vi "Write Result.vi"(8 "error in (no error)":errorcluster, 10 "Result":dbl, 11 "DBL Result Class in":refnum<class "DBL Result Class.lvclass">) -> (0 "error out":errorcluster, 3 "DBL Result Class out":refnum<class "DBL Result Class.lvclass">)   [LabVIEW 2018, in "DBL Result Class.lvclass"]
uses:
  DBL Result Class.lvclass
  DBL Result Class.lvclass/DBL Result Class.ctl
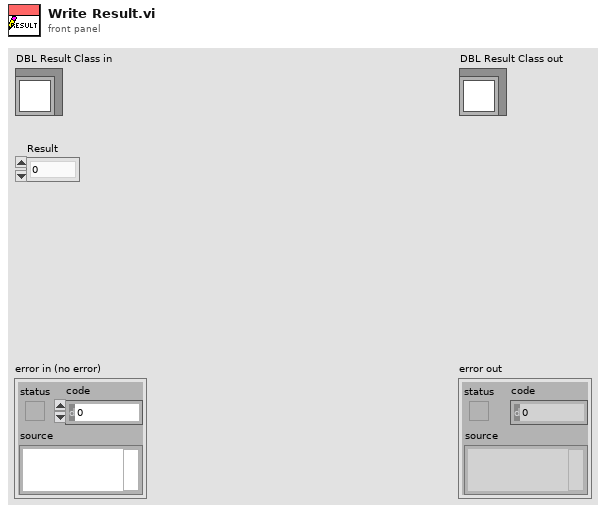
[diagram p1: front panel]
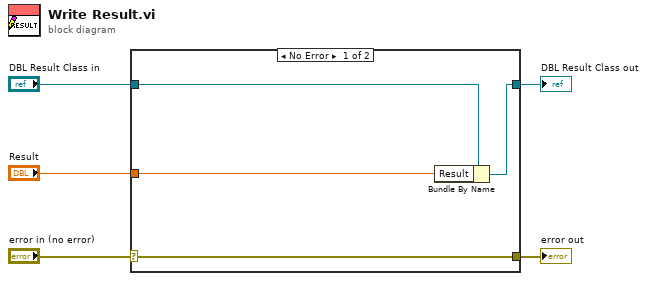
[diagram p0: block diagram]
diagram:
  n1 = case shown="No Error" "error in (no error)" {
    selector: "error in (no error)" -> [w9 w10]
    tunnel: [w9 w10] -> w4
    tunnel: [w7 w11] -> w2
    tunnel: "DBL Result Class in" -> [w8 w11]
    tunnel: "Result" -> [w6 _]
    frame No Error {
      n2 = Bundle By Name(cluster=w8, "Result"=w6) -> (w7:refnum<class "DBL Result Class.lvclass">)
    }
    frame Error {
    }
  }
  "error out" <- w4
  "DBL Result Class out" <- w2
